vi "evaluateGenerateXML.vi"(8 "error in":errorcluster, 9 "Input Data":variant, 11 "reference in":refnum<class "EasyXML_XML_Subset_Source_Tests.lvclass">) -> (0 "error out":errorcluster, 1 "XML String":string, 3 "reference out":refnum<class "EasyXML_XML_Subset_Source_Tests.lvclass">)   [LabVIEW 2013, in "EasyXML_XML_Subset_Source_Tests.lvclass"]
uses:
  EasyXML_XML_Subset_Source_Tests.lvclass
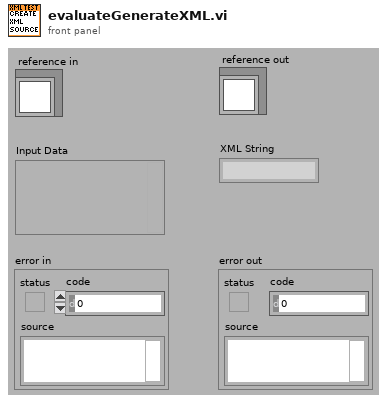
[diagram p1: front panel]
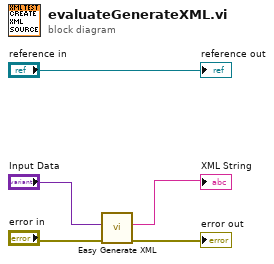
[diagram p0: block diagram]
diagram:
  n1 = call "Easy Generate XML.vi"("error in (no error)"="error in", "LabVIEW Data"="Input Data") -> ("error out"=→"error out":errorcluster, "XML String"=→"XML String":string)  [unwired: 8 in]
  "reference out" <- "reference in"
